vi "changeState.vi"(8 "error in (no error)":errorcluster, 10 "DetailedStates":T1=enum."StandbyState", 11 "Model in":refnum<class "Model.lvclass">) -> (0 "error out":errorcluster, 3 "Model out":refnum<class "Model.lvclass">)   [LabVIEW 2016, in "Model.lvclass"]
uses:
  Model.lvclass
  DataTypes/Topics/Parts/DetailedStates.ctl
  DataTypes/Topics/Parts/SummaryStates.ctl
  Model.lvclass/Model.ctl
  DataTypes/Topics/M1M3SupportTopics.lvlib
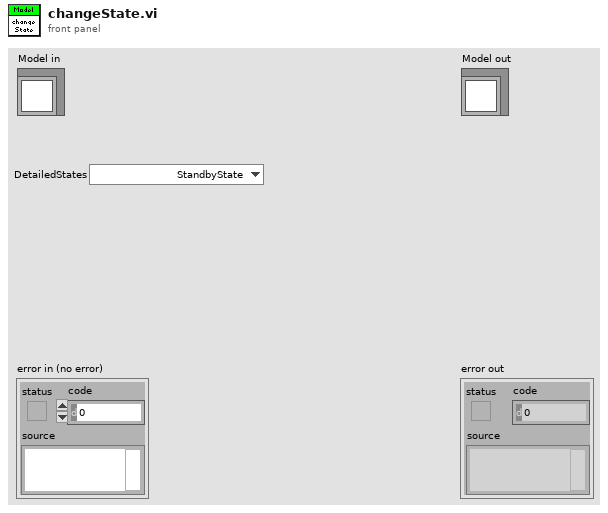
[diagram p1: front panel]
types:
  T1 = typedef "M1M3SupportTopics.lvlib/DetailedStates.ctl" = enum16{"OfflineState", "InitialState", "StandbyState", "DisabledState", "ParkedState", "FaultState", "ParkedMaintenanceState", "ActiveMaintenanceState"}
  T2 = typedef "M1M3SupportTopics.lvlib/SummaryStates.ctl" = enum16{"OfflineState", "StandbyState", "DisabledState", "EnabledState", "FaultState"}
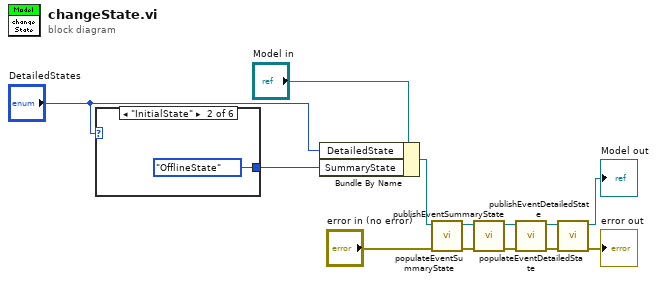
[diagram p0: block diagram]
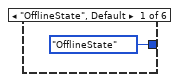
[diagram p2: hidden frame]
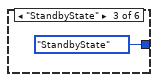
[diagram p3: hidden frame]
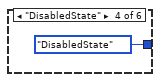
[diagram p4: hidden frame]
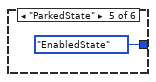
[diagram p5: hidden frame]
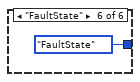
[diagram p6: hidden frame]
diagram:
  n1 = case shown="\"InitialState\"" "DetailedStates" {
    tunnel: [SummaryStates."OfflineState" ("SummaryState") SummaryStates."OfflineState" ("SummaryState") SummaryStates."StandbyState" ("SummaryState") SummaryStates."DisabledState" ("SummaryState") SummaryStates."EnabledState" ("SummaryState") SummaryStates."FaultState" ("SummaryState")] -> w11
    frame "OfflineState", Default {
    }
    frame "InitialState" {
    }
    frame "StandbyState" {
    }
    frame "DisabledState" {
    }
    frame "ParkedState" {
    }
    frame "FaultState" {
    }
  }
  n2 = Bundle By Name(cluster="Model in", "DetailedState"="DetailedStates", "SummaryState"=w11) -> (w10:refnum<class "Model.lvclass">)
  n3 = call "populateEventSummaryState.vi"("error in (no error)"="error in (no error)", "Model in"=w10) -> ("error out"=w7:errorcluster, "Model out"=w9:refnum<class "Model.lvclass">)  [unwired: 8 in]
  n4 = call "publishEventSummaryState.vi"("error in (no error)"=w7, "Model in"=w9) -> ("error out"=w3:errorcluster, "Model out"=w6:refnum<class "Model.lvclass">)  [unwired: 8 in]
  n5 = call "populateEventDetailedState.vi"("error in (no error)"=w3, "Model in"=w6) -> ("error out"=w2:errorcluster, "Model out"=w5:refnum<class "Model.lvclass">)  [unwired: 8 in]
  n6 = call "publishEventDetailedState.vi"("error in (no error)"=w2, "Model in"=w5) -> ("error out"=→"error out":errorcluster, "Model out"=→"Model out":refnum<class "Model.lvclass">)  [unwired: 8 in]
